vi "Basic Control.vi"() -> ()   [LabVIEW 2019, in "ACSVcontrol-driver.lvlib"]
doc: "This VI gives basic control to the PJVS system. Intended as an example or for manual testing."
uses:
  ACSVcontrol-driver.lvlib
  Type Definitions/Multiplexer.ctl
  Type Definitions/Waveform.ctl
  Type Definitions/Sensors Data.ctl
  Type Definitions/PJVS Voltages.ctl
  Type Definitions/Timeouts.ctl
  Type Definitions/Debug status.ctl
  <vilib>/Utility/miscctls.llb/LVRowAndColumnUnsignedTypeDef.ctl
  <vilib>/Utility/miscctls.llb/LVRowAndColumnTypeDef.ctl
panel:
  in  "Abort":bool
  in  "Tab Control":T1(tab)
  in  "Simulation mode":bool caption="Simulation mode\n\nIf set, driver is switched into simulation mode.\nNo tcp connection is required and output data\nare generated randomly."
  in  "Timeouts":T2={"TCP Read & Write (ms)"=7000, "Sensors readout"=5000, "PJVS setup"=10000, "Nullmeter readout"=5000, "Multiplexer setup"=3000, "57XX setup"=15000, "Generator setup"=5000, "Synthesizer setup"=3000, "Sampler readout"=10000}
  in  "IP address:port":string="192.168.1.2:31180"
  in  "update timeouts":bool
  out "Power ()":dbl
  out "Synth frequency":dbl caption="Frequency (Hz)" format="%#_12p"
  in  "On/Off":bool
  in  "synth":bool
  out "PJVS Voltages":T3={"DC Voltage (S)"=nan, "AC Josephson Voltage RMS (V)"=nan, "Number of steps"=-1, "AC Voltages (V)"=[]} {"AC Josephson Voltage RMS (V)" format="%#_10g"; "DC Voltage (S)" format="%#_10g"}
  in  "Samples (2 - 256)":i32=20 min=2 max=256
  in  "Waveform (Sinewave)":T4
  in  "Trim current (A) (+- 0.002)":dbl
  in  "PJVS frequency":dbl=1000.0 caption="Frequency  (0, 0.5 - 10e3)"
  in  "PJVS voltage":dbl=0.1 caption="Voltage (V) \n(DC: +- 10.1, AC: 0 - 7.2)"
  in  "Waveform (F) (F:Sine, T:Square)":bool
  in  "Init (F)":bool=TRUE
  in  "Generator phase":dbl=170.4 caption="Phase (0 °) (0 - 359.99)"
  in  "Generator frequency":dbl=1000.0 caption="Frequency (125 Hz) (0.01 - 50e6)"
  in  "Generator amplitude":dbl=2.5 caption="Voltage (2.5 V pp) (0.1 - 5)"
  in  "Generator":bool
  in  "mux":bool
  in  "Filter (F)":bool
  in  "ShortNano (F)":bool
  in  "AC (F) (F:Nano, T:Digitizer)":bool
  in  "Multiplexer (Short DC Nano / Voltmeter)":T5=enum."Short AC Sampler"
  in  "Trigger Slope (F)":bool
  out "No of Sampler Results":i32
  out "Sampler Mean (V)":dbl format="%#_9g"
  out "Sampler Std. Dev. (V)":dbl
  in  "Sampler":bool
  out "Sampler Results (V)":dbl[](array[numeric]) format="%#_9g"
  in  "Meas. Time (1 s) (0.01 - 10)":dbl=0.1
  in  "Loops (10) (1 - 1000)":i32=1
  in  "Vertical Range (V)":dbl=5.0
  in  "Result as Mean?":bool=TRUE
  in  "sensors":bool
  out "Nulldet. Results (V)":dbl[](array[numeric]) format="%#_9g"
  in  "Readings":i32=1
  in  "nulldetector":bool
  out "No of Nulldet. Results":i32
  in  "PJVS":bool
  out "Sensors Data":T6={"Temperature (°C)"=nan, "Barometric Pressure (mbar)"=nan, "Humidity (%)"=nan, "Temperature Cooler (K)"=nan}
  in  "57XX":bool
  in  "Phase Lock (T)":bool=TRUE
  in  "Current (F)":bool
  in  "ext. Guard (F)":bool
  in  "57XX amplitude":dbl=0.1 caption="Voltage/Current (V, V rms, A) (1)"
  in  "57XX frequency":dbl=1000.0 caption="Frequency (125 Hz) (0, 10 - 10e3)"
  out "Waveform Graph":dbl[](graph)
  out "PJVS waveform":dbl[](graph)
  in  "Interlock frequencies":bool=TRUE caption="Change of one freuqency\nchanges also numbers for:\n- PJVS\n- Generator\n- 57XX\n(does not send any\ncommands)"
  in  "export table to excell":bool
  in  "Clear table":bool
  out "Debug data":string[][](table)
  in  "Debug mode":bool
  in  "status":bool
  out "last error":errorcluster
  out "Last Status:":string
  in  "quit":bool
  # "Example for ACSVcontrol-driver"
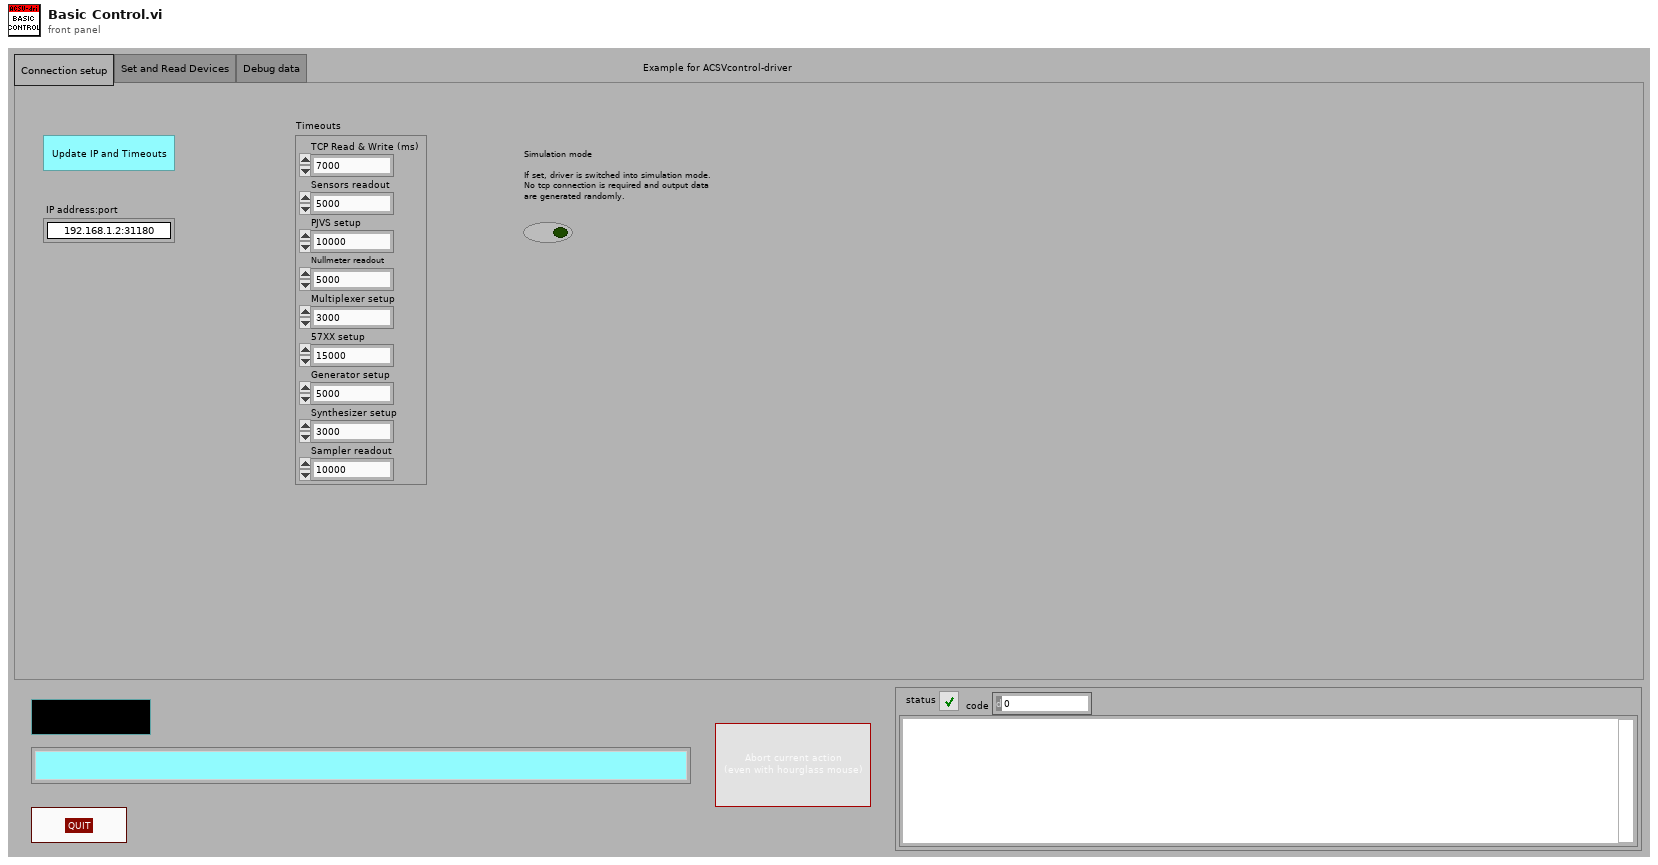
[diagram p1: front panel]
types:
  T1 = enum32{"Connection setup", "Set and Read Devices", "Debug data"}
  T2 = typedef "ACSVcontrol-driver.lvlib/Timeouts.ctl" = cluster{"TCP Read & Write (ms)":i32, "Sensors readout":i32, "PJVS setup":i32, "Nullmeter readout":i32, "Multiplexer setup":i32, "57XX setup":i32, "Generator setup":i32, "Synthesizer setup":i32, "Sampler readout":i32}
  T3 = typedef "ACSVcontrol-driver.lvlib/PJVS Voltages.ctl" = cluster{"DC Voltage (S)":dbl, "AC Josephson Voltage RMS (V)":dbl, "Number of steps":i32, "AC Voltages (V)":dbl[]}
  T4 = typedef "ACSVcontrol-driver.lvlib/Waveform.ctl" = enum16{"Sinewave", "Triangle", "Sawtooth", "Rectangle", "Arbitrary"}
  T5 = typedef "ACSVcontrol-driver.lvlib/Multiplexer.ctl" = enum16{"Short DC Nano / Voltmeter", "Short AC Sampler", "Short Switch DC (JVS->Nano)", "Short Switch AC (JVS->Digit)", "JVS-Voltmeter", "Channel A positive", "Channel A negative", "Channel B positive", "Channel B negative", "Channel C positive", "Channel C negative", "Nulldetector-Channel A+", "Nulldetector-Channel A-", "Nulldetector-Channel B+", "Nulldetector-Channel B-", "Nulldetector-Channel C+", "Nulldetector-Channel C-", "ext.Voltmeter-Channel A+", "ext.Voltmeter-Channel A-", "ext.Voltmeter-Channel B+", "ext.Voltmeter-Channel B-", "ext.Voltmeter-Channel C+", "ext.Voltmeter-Channel C-"}
  T6 = typedef "ACSVcontrol-driver.lvlib/Sensors Data.ctl" = cluster{"Temperature (°C)":dbl, "Barometric Pressure (mbar)":dbl, "Humidity (%)":dbl, "Temperature Cooler (K)":dbl}
  T7 = typedef "LVRowAndColumnUnsignedTypeDef.ctl" = cluster{"Row":u32, "Column":u32}
  T8 = enum8{"Enabled", "Disabled", "Disabled and Grayed Out"}
  T9 = typedef "ACSVcontrol-driver.lvlib/Debug status.ctl" = enum16{"No change", "Off", "On"}
  T10 = typedef "LVRowAndColumnTypeDef.ctl" = cluster{"Row":i32, "Column":i32}
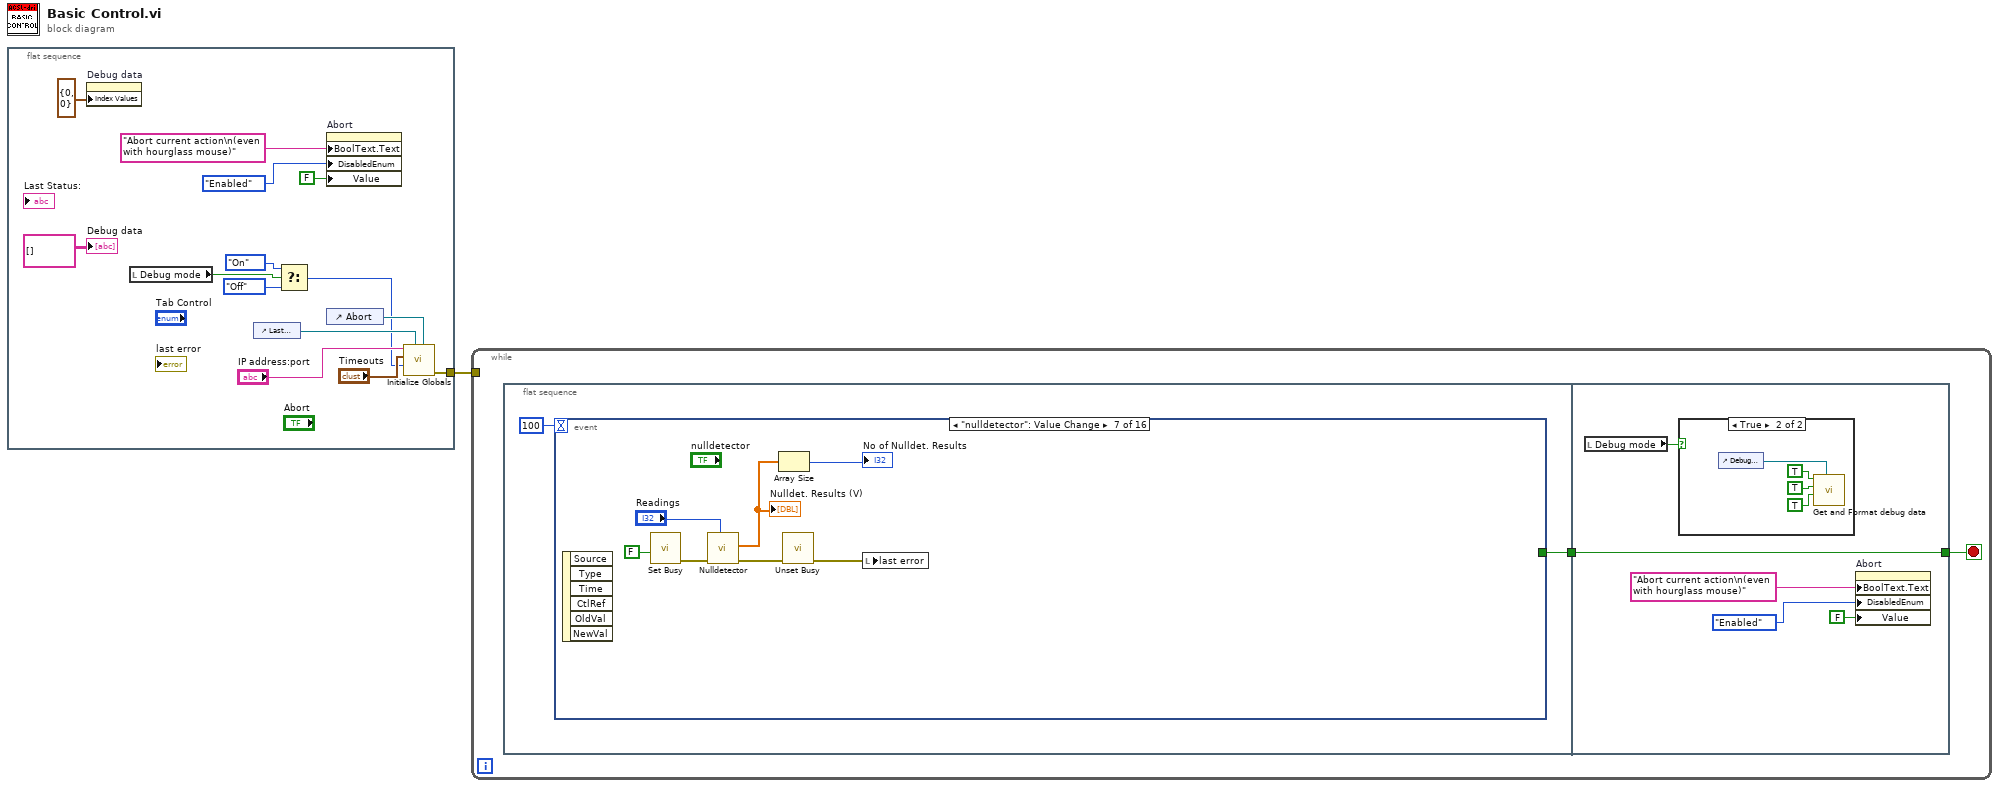
[diagram p0: block diagram]
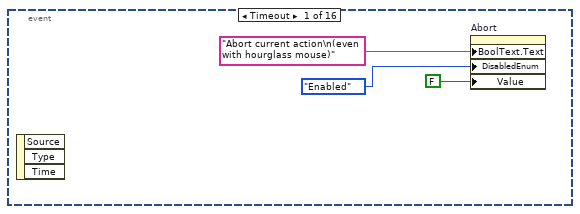
[diagram p2: hidden frame]
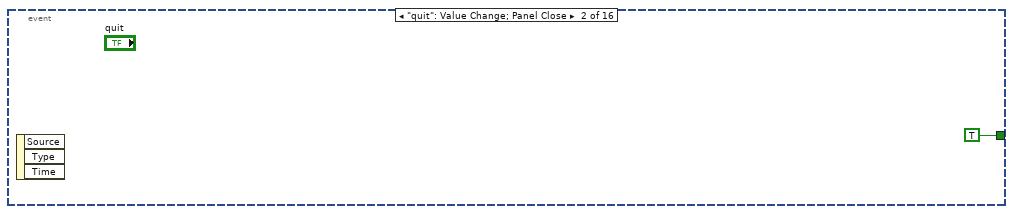
[diagram p3: hidden frame]
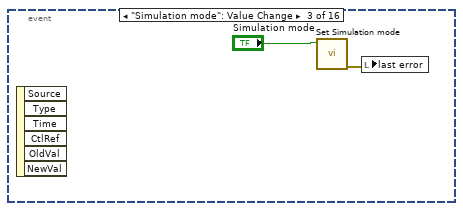
[diagram p4: hidden frame]
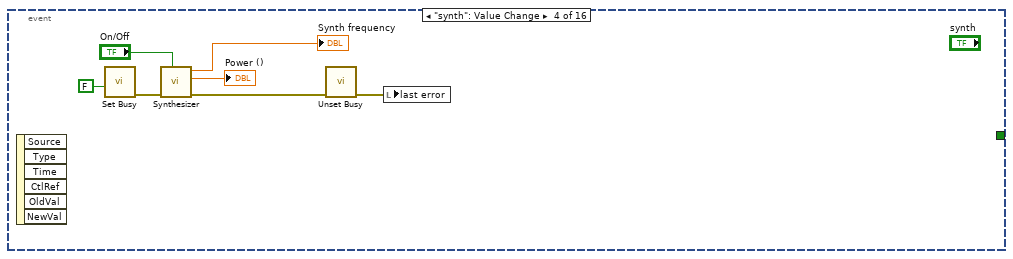
[diagram p5: hidden frame]
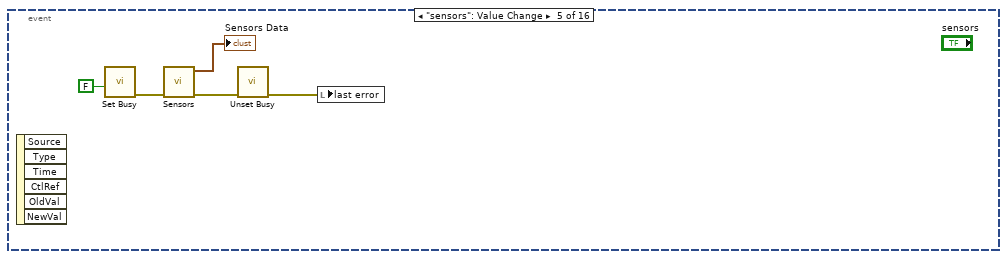
[diagram p6: hidden frame]
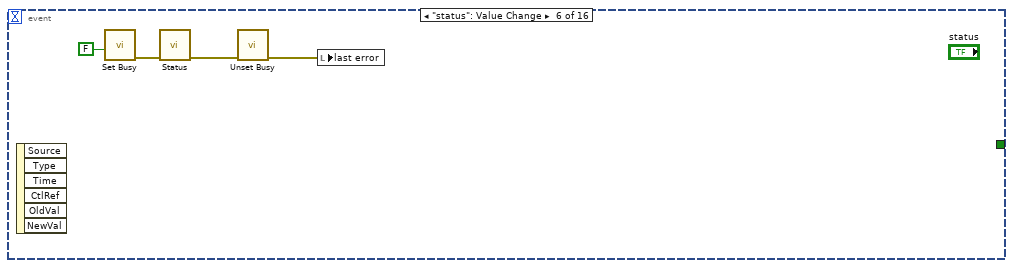
[diagram p7: hidden frame]
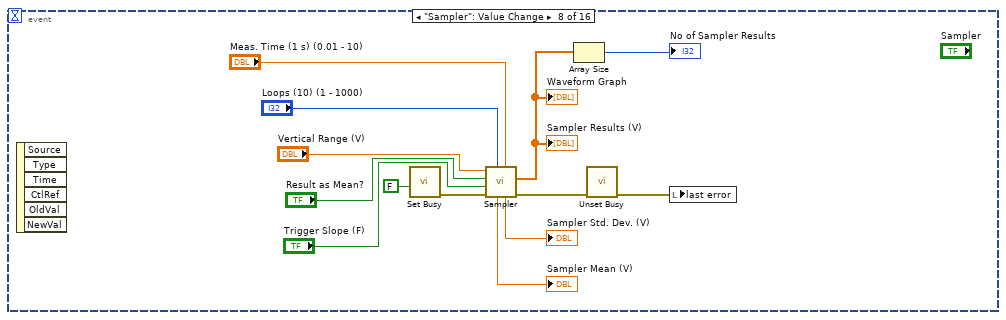
[diagram p8: hidden frame]
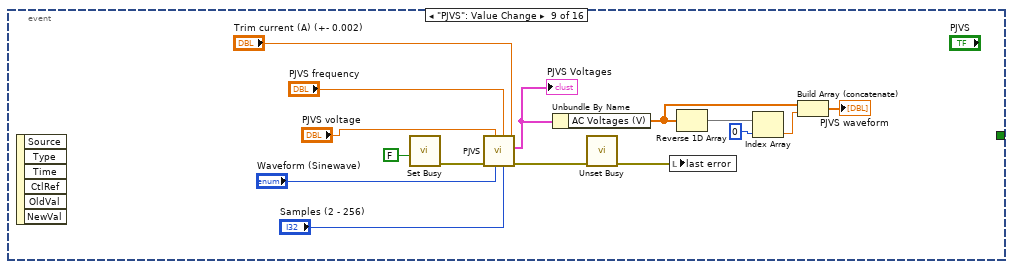
[diagram p9: hidden frame]
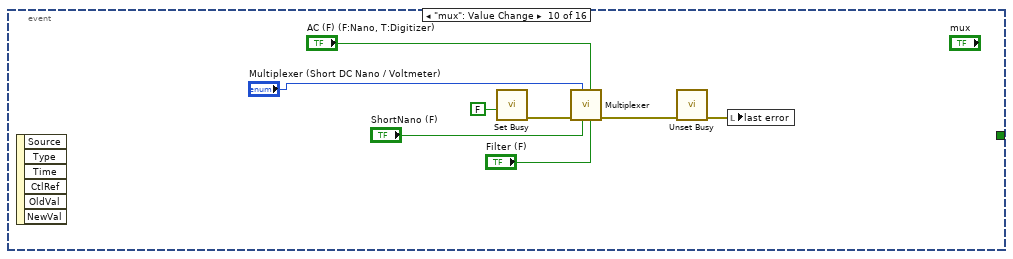
[diagram p10: hidden frame]
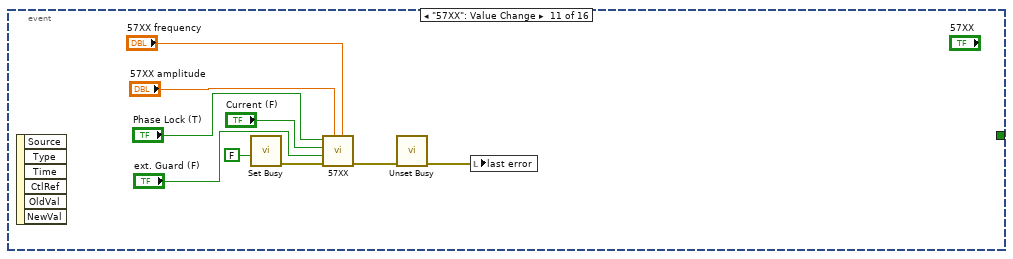
[diagram p11: hidden frame]
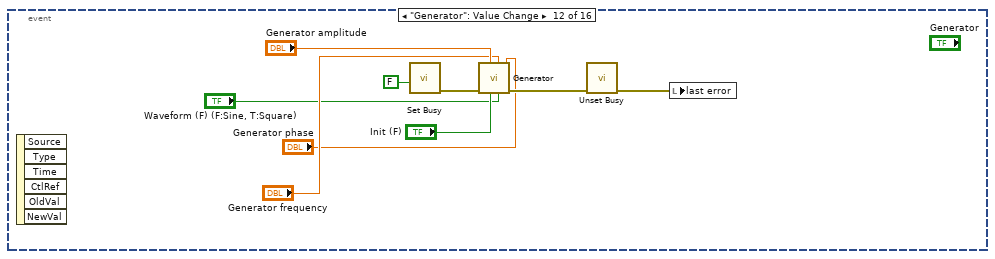
[diagram p12: hidden frame]
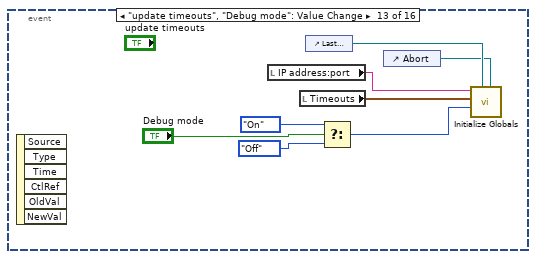
[diagram p13: hidden frame]
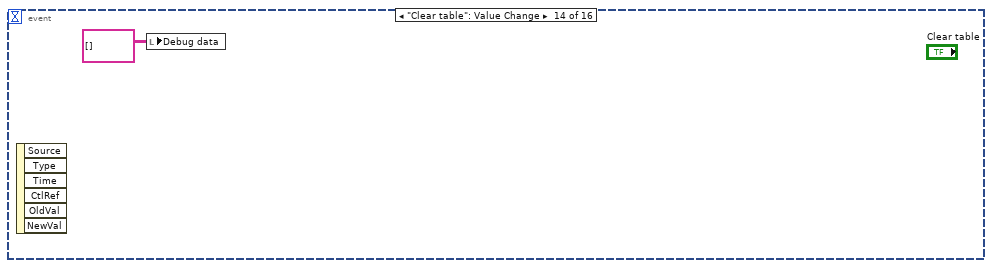
[diagram p14: hidden frame]
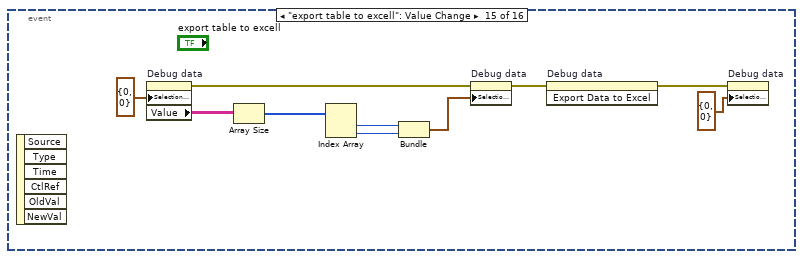
[diagram p15: hidden frame]
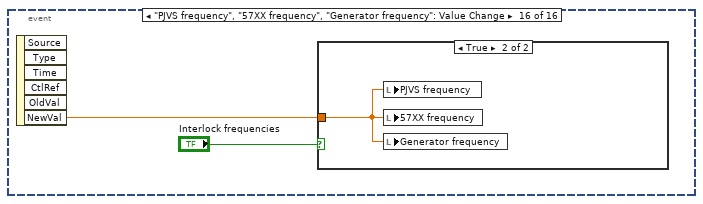
[diagram p16: hidden frame]
diagram:
  n1 = flat-sequence {
    tunnel: [w11] -> w1
    frame #0 {
      n2 = property on="Debug data" class="Tbl (strict)"("Index Values"=T7 {"Row"=0, "Column"=0}) -> ()  [unwired: 2 in, 2 out]
      n3 = local read "Debug mode"() -> (w10:bool)
      n4 = control-ref of="Last Status:"() -> (w13:refnum<vi>)
      n5 = Select(t=Debug_status."On" ("Debug mode"), s=w10, f=Debug_status."Off" ("Debug mode")) -> (s? t:f=w8:T9)
      n6 = property on="Abort" class="Bool (strict)"("BoolText.Text"="Abort current action\n(even with hourglass mouse)" ("Boolean Text.Text"), "DisabledEnum"=T8."Enabled" ("Disabled"), "Value"=FALSE ("Abort")) -> ()  [unwired: 2 in, 2 out]
      n7 = control-ref of="Abort"() -> (w15:refnum<vi>)
      n8 = call "Initialize Globals.vi"("Abort Refnum"=w15, "Status Refnum"=w13, "Debug mode"=w8, "Timeouts"="Timeouts", "IP address:port (0.0.0.0:0000)"="IP address:port") -> ("error out"=w11:errorcluster)  [unwired: 1 in, 5 out]
      "Debug data" <- string[][] [] ("Debug data")
    }
  }
  n9 = while {
    tunnel: w1 -> [_]
    stop <- w17 stop-if-true
    n10 = flat-sequence {
      tunnel: [w19] -> w16
      tunnel: [w129] -> w17
      tunnel: w16 -> [w129]
      frame #0 {
        n11 = event shown="[6] \"nulldetector\": Value Change" {
          selector: _ -> [_ _ _ _ _ _ _ _ _ _ _ _ _ _ _ _]
          dyn-events: _ -> [_ _ _ _ _ _ _ _ _ _ _ _ _ _ _ _]
          timeout: 100 -> [_ _ _ _ _ _ _ _ _ _ _ _ _ _ _ _]
          tunnel: [_ TRUE _ _ _ _ _ _ _ _ _ _ _ _ _ _] -> w19
          event Timeout {
            n12 = event-data() -> ()  [unwired: 1 in, 3 out]
            n13 = property on="Abort" class="Bool (strict)"("BoolText.Text"="Abort current action\n(even with hourglass mouse)" ("Boolean Text.Text"), "DisabledEnum"=T8."Enabled" ("Disabled"), "Value"=FALSE ("Abort")) -> ()  [unwired: 2 in, 2 out]
          }
          event "quit": Value Change; Panel Close {
            n14 = event-data() -> ()  [unwired: 1 in, 3 out]
          }
          event "Simulation mode": Value Change {
            n15 = event-data() -> ()  [unwired: 1 in, 6 out]
            n16 = call "Set Simulation mode.vi"("Simulation mode (T)"="Simulation mode") -> ("error out (passthrough)"=w24:errorcluster)  [unwired: 10 in]
            n17 = local write "last error"(w24) -> ()
          }
          event "synth": Value Change {
            n18 = event-data() -> ()  [unwired: 1 in, 6 out]
            n19 = call <vilib>:"Set Busy.vi"("disable click? (T)"=FALSE) -> ("error out"=w29:errorcluster)  [unwired: 9 in, 1 out]
            n20 = call "Synthesizer.vi"("Status (F) (F: Off, T: On)"="On/Off", "error in (no error)"=w29) -> ("error out"=w28:errorcluster, "Power"=→"Power ()":dbl, "Frequency (GHz)"=→"Synth frequency":dbl)  [unwired: 7 in]
            n21 = call <vilib>:"Unset Busy.vi"("error in (no error)"=w28) -> ("error out"=w27:errorcluster)  [unwired: 10 in]
            n22 = local write "last error"(w27) -> ()
          }
          event "sensors": Value Change {
            n23 = event-data() -> ()  [unwired: 1 in, 6 out]
            n24 = call <vilib>:"Set Busy.vi"("disable click? (T)"=FALSE) -> ("error out"=w36:errorcluster)  [unwired: 9 in, 1 out]
            n25 = call "Sensors.vi"("error in (no error)"=w36) -> ("error out"=w35:errorcluster, "Sensors Data"=→"Sensors Data":T6)  [unwired: 9 in]
            n26 = call <vilib>:"Unset Busy.vi"("error in (no error)"=w35) -> ("error out"=w34:errorcluster)  [unwired: 10 in]
            n27 = local write "last error"(w34) -> ()
          }
          event "status": Value Change {
            n28 = event-data() -> ()  [unwired: 1 in, 6 out]
            n29 = call <vilib>:"Set Busy.vi"("disable click? (T)"=FALSE) -> ("error out"=w41:errorcluster)  [unwired: 9 in, 1 out]
            n30 = call "Status.vi"("error in (no error)"=w41) -> ("error out"=w39:errorcluster)  [unwired: 7 in, 3 out]
            n31 = call <vilib>:"Unset Busy.vi"("error in (no error)"=w39) -> ("error out"=w40:errorcluster)  [unwired: 10 in]
            n32 = local write "last error"(w40) -> ()
          }
          event "nulldetector": Value Change {
            n33 = event-data() -> ()  [unwired: 1 in, 6 out]
            n34 = call <vilib>:"Set Busy.vi"("disable click? (T)"=FALSE) -> ("error out"=w46:errorcluster)  [unwired: 9 in, 1 out]
            n35 = call "Nulldetector.vi"("Readings (10)"="Readings", "error in (no error)"=w46) -> ("error out"=w47:errorcluster, "Voltages (V)"=w42:dbl[])  [unwired: 7 in, 1 out]
            "Nulldet. Results (V)" <- w42
            n36 = Array Size(array=w42) -> (size(s)=→"No of Nulldet. Results":i32)
            n37 = call <vilib>:"Unset Busy.vi"("error in (no error)"=w47) -> ("error out"=w45:errorcluster)  [unwired: 10 in]
            n38 = local write "last error"(w45) -> ()
          }
          event "Sampler": Value Change {
            n39 = event-data() -> ()  [unwired: 1 in, 6 out]
            n40 = call <vilib>:"Set Busy.vi"("disable click? (T)"=FALSE) -> ("error out"=w59:errorcluster)  [unwired: 9 in, 1 out]
            n41 = call "Sampler.vi"("Meas. Time (1 s) (0.01 - 10)"="Meas. Time (1 s) (0.01 - 10)", "Loops (10) (1 - 1000)"="Loops (10) (1 - 1000)", "error in (no error)"=w59, "Trigger Slope (F)"="Trigger Slope (F)", "Result as Mean? (F)"="Result as Mean?", "Vertical Range (V)"="Vertical Range (V)") -> ("error out"=w58:errorcluster, "RMS Voltages (V)"=w51:dbl[], "Std. Dev. (V)"=→"Sampler Std. Dev. (V)":dbl, "Mean (V)"=→"Sampler Mean (V)":dbl)  [unwired: 2 in]
            "Sampler Results (V)" <- w51
            "Waveform Graph" <- w51
            n42 = Array Size(array=w51) -> (size(s)=→"No of Sampler Results":i32)
            n43 = call <vilib>:"Unset Busy.vi"("error in (no error)"=w58) -> ("error out"=w61:errorcluster)  [unwired: 10 in]
            n44 = local write "last error"(w61) -> ()
          }
          event "PJVS": Value Change {
            n45 = event-data() -> ()  [unwired: 1 in, 6 out]
            n46 = call <vilib>:"Set Busy.vi"("disable click? (T)"=FALSE) -> ("error out"=w71:errorcluster)  [unwired: 9 in, 1 out]
            n47 = call "PJVS.vi"("Trim current (A) (+- 0.002)"="Trim current (A) (+- 0.002)", "Samples (2) (2 - 256)"="Samples (2 - 256)", "Frequency  (0 Hz) (0, 0.5 - 10e3)"="PJVS frequency", "Waveform (Sinewave)"="Waveform (Sinewave)", "Voltage (0 V DC/RMS) (DC: +- 10.1, AC: 0 - 7.2)"="PJVS voltage", "error in (no error)"=w71) -> ("error out"=w70:errorcluster, "PJVS Voltages"=w67:T3)  [unwired: 4 in]
            "PJVS Voltages" <- w67
            n48 = Unbundle By Name(w67) -> ("AC Voltages (V)"=w62:dbl[])
            n49 = call <vilib>:"Unset Busy.vi"("error in (no error)"=w70) -> ("error out"=w69:errorcluster)  [unwired: 10 in]
            n50 = local write "last error"(w69) -> ()
            n51 = Reverse 1D Array(array=w62) -> (reversed array=w64:dbl[])
            n52 = Index Array(array=w64, index=0) -> (element=w65:dbl)
            n53 = Build Array (concatenate)(w62, w65) -> (→"PJVS waveform":dbl[])
          }
          event "mux": Value Change {
            n54 = event-data() -> ()  [unwired: 1 in, 6 out]
            n55 = call <vilib>:"Set Busy.vi"("disable click? (T)"=FALSE) -> ("error out"=w80:errorcluster)  [unwired: 9 in, 1 out]
            n56 = call "Multiplexer.vi"("Filter (F)"="Filter (F)", "AC (F) (F:Nano, T:Digitizer)"="AC (F) (F:Nano, T:Digitizer)", "ShortNano (F)"="ShortNano (F)", "Multiplexer (Short DC Nano / Voltmeter)"="Multiplexer (Short DC Nano / Voltmeter)", "error in (no error)"=w80) -> ("error out"=w79:errorcluster)  [unwired: 6 in]
            n57 = call <vilib>:"Unset Busy.vi"("error in (no error)"=w79) -> ("error out"=w78:errorcluster)  [unwired: 10 in]
            n58 = local write "last error"(w78) -> ()
          }
          event "57XX": Value Change {
            n59 = event-data() -> ()  [unwired: 1 in, 6 out]
            n60 = call <vilib>:"Set Busy.vi"("disable click? (T)"=FALSE) -> ("error out"=w88:errorcluster)  [unwired: 9 in, 1 out]
            n61 = call "57XX.vi"("Frequency (125 Hz) (0, 10 - 10e3)"="57XX frequency", "Voltage/Current (V, V rms, A) (1)"="57XX amplitude", "error in (no error)"=w88, "ext. Guard (F)"="ext. Guard (F)", "Current (F)"="Current (F)", "Phase Lock (T)"="Phase Lock (T)") -> ("error out"=w87:errorcluster)  [unwired: 5 in]
            n62 = call <vilib>:"Unset Busy.vi"("error in (no error)"=w87) -> ("error out"=w86:errorcluster)  [unwired: 10 in]
            n63 = local write "last error"(w86) -> ()
          }
          event "Generator": Value Change {
            n64 = event-data() -> ()  [unwired: 1 in, 6 out]
            n65 = call <vilib>:"Set Busy.vi"("disable click? (T)"=FALSE) -> ("error out"=w100:errorcluster)  [unwired: 9 in, 1 out]
            n66 = call "Generator.vi"("Phase (0 °) (0 - 359.99)"="Generator phase", "Waveform (F) (F:Sine, T:Square)"="Waveform (F) (F:Sine, T:Square)", "Frequency (125 Hz) (0.01 - 50e6)"="Generator frequency", "Init (F)"="Init (F)", "Voltage (2.5 V pp) (0.1 - 5)"="Generator amplitude", "error in (no error)"=w100) -> ("error out"=w101:errorcluster)  [unwired: 5 in]
            n67 = call <vilib>:"Unset Busy.vi"("error in (no error)"=w101) -> ("error out"=w102:errorcluster)  [unwired: 10 in]
            n68 = local write "last error"(w102) -> ()
          }
          event "update timeouts", "Debug mode": Value Change {
            n69 = event-data() -> ()  [unwired: 1 in, 6 out]
            n70 = local read "IP address:port"() -> (w107:string)
            n71 = local read "Timeouts"() -> (w108:T2)
            n72 = control-ref of="Last Status:"() -> (w110:refnum<vi>)
            n73 = Select(t=Debug_status."On" ("Debug mode"), s="Debug mode", f=Debug_status."Off" ("Debug mode")) -> (s? t:f=w103:T9)
            n74 = control-ref of="Abort"() -> (w109:refnum<vi>)
            n75 = call "Initialize Globals.vi"("Abort Refnum"=w109, "Status Refnum"=w110, "Debug mode"=w103, "Timeouts"=w108, "IP address:port (0.0.0.0:0000)"=w107) -> ()  [unwired: 1 in, 6 out]
          }
          event "Clear table": Value Change {
            n76 = event-data() -> ()  [unwired: 1 in, 6 out]
            n77 = local write "Debug data"(string[][] [] ("Debug data")) -> ()
          }
          event "export table to excell": Value Change {
            n78 = event-data() -> ()  [unwired: 1 in, 6 out]
            n79 = property on="Debug data" class="Tbl (strict)"("Selection Start"=T10 {"Row"=0, "Column"=0}) -> (error out=w115:errorcluster, "Value"=w120:string[][])  [unwired: 2 in, 1 out]
            n80 = Array Size(array=w120) -> (size(s)=w119:i32[])
            n81 = Index Array(array=w119) -> (element #1=w118:i32, element #2=w117:i32)  [unwired: 2 in]
            n82 = Bundle(w118, w117) -> (w116:cluster{i32, i32})  [unwired: 1 in]
            n83 = property on="Debug data" class="Tbl (strict)"(error in=w115, "Selection Size"=w116) -> (error out=w114:errorcluster)  [unwired: 1 in, 1 out]
            n84 = invoke on="Debug data" class="Tbl (strict)" method="Export Data to Excel"(error in=w114) -> (error out=w113:errorcluster)  [unwired: 2 in, 2 out]
            n85 = property on="Debug data" class="Tbl (strict)"(error in=w113, "Selection Size"=T10 {"Row"=0, "Column"=0}) -> ()  [unwired: 1 in, 2 out]
          }
          event "PJVS frequency", "57XX frequency", "Generator frequency": Value Change {
            n86 = event-data() -> ("NewVal"=w123:dbl)  [unwired: 1 in, 5 out]
            n87 = case shown="True" "Interlock frequencies" {
              tunnel: w123 -> [_ w124]
              frame False {
              }
              frame True {
                n88 = local write "PJVS frequency"(w124) -> ()
                n89 = local write "57XX frequency"(w124) -> ()
                n90 = local write "Generator frequency"(w124) -> ()
              }
            }
          }
        }
      }
      frame #1 {
        n91 = local read "Debug mode"() -> (w128:bool)
        n92 = case shown="True" w128 {
          frame False {
          }
          frame True {
            n93 = control-ref of="Debug data"() -> (w133:refnum<vi>)
            n94 = call "Get and Format debug data.vi"("Table Control refnum"=w133, "Update table position?"=TRUE, "Format debug data?"=TRUE, "Empty debug data?"=TRUE) -> ()  [unwired: 6 in, 2 out]
          }
        }
        n95 = property on="Abort" class="Bool (strict)"("BoolText.Text"="Abort current action\n(even with hourglass mouse)" ("Boolean Text.Text"), "DisabledEnum"=T8."Enabled" ("Disabled"), "Value"=FALSE ("Abort")) -> ()  [unwired: 2 in, 2 out]
      }
    }
  }
